vi "InitPVCAMGetCamNames.vi"() -> (0 "error out":errorcluster, 2 "Array":string[](array[string]), 3 "number of cameras":i32)   [LabVIEW 2021]
panel:
  in  "error in (no error)":errorcluster
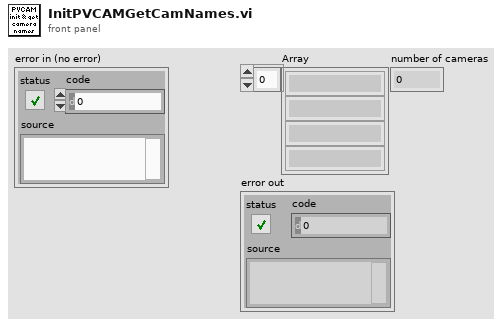
[diagram p1: front panel]
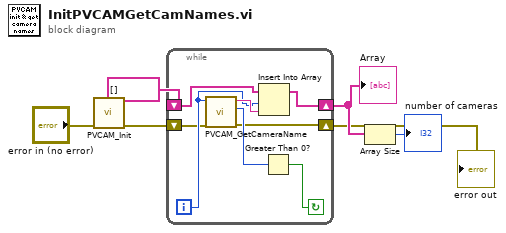
[diagram p0: block diagram]
diagram:
  n1 = call "PVCAM_Init.vi"("error in (no error)"="error in (no error)") -> ("error out"=w4:errorcluster)  [unwired: 9 in, 1 out]
  n2 = while {
    shift-right: [w12] -> w3
    shift-left: string[] [] -> [w9]
    shift-right: [w7] -> w1
    shift-left: w4 -> [w8]
    i -> [w10]
    stop <- w13 continue-if-true
    n3 = call "PVCAM_GetCameraName.vi"("error in (no error)"=w8, "index in"=w10) -> ("error out"=w7:errorcluster, "return out"=w14:i16, "string"=w11:string)  [unwired: 6 in, 1 out]
    n4 = Insert Into Array(array=w9, index=w10, new element=w11) -> (w12:string[])
    n5 = Greater Than 0?(x=w14) -> (x > 0?=w13:bool)
  }
  "Array" <- w3
  "error out" <- w1
  n6 = Array Size(array=w3) -> (size(s)=→"number of cameras":i32)
